vi "孔径结果转换.vi"(11 "Fitted Circle (Find Circular Edge 1)":T1 {"Average SNR (dB)" format="%.2f"; "Average Strength" format="%.2f"; "Roundness (Real-World)" format="%.2f"; "Radius (Real-World)" format="%.2f"; "Center (Real-World)"."Y" format="%.2f"; "Center (Real-World)"."X" format="%.2f"; "Radius (Pixels)" format="%.2f"; "Center (Pixels)"."Y" format="%.2f"; "Center (Pixels)"."X" format="%.2f"}) -> (3 "x+y":dbl format="%#_3f")   [LabVIEW 2017]
uses:
  Global System.vi
panel:
  out "F-格式字符串":string
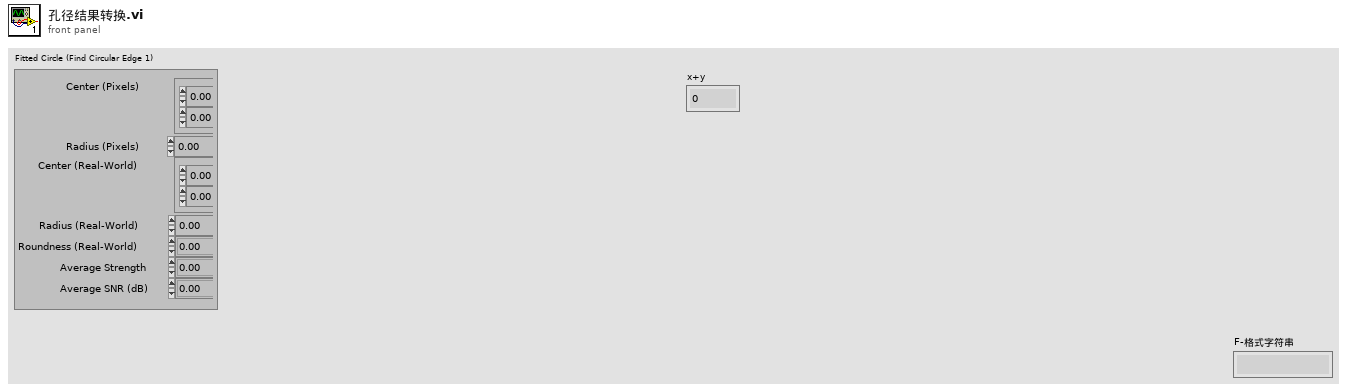
[diagram p1: front panel]
types:
  T1 = cluster{"Center (Pixels)":cluster{"X":sgl, "Y":sgl}, "Radius (Pixels)":dbl, "Center (Real-World)":cluster{"X":sgl, "Y":sgl}, "Radius (Real-World)":dbl, "Roundness (Real-World)":dbl, "Average Strength":dbl, "Average SNR (dB)":dbl}
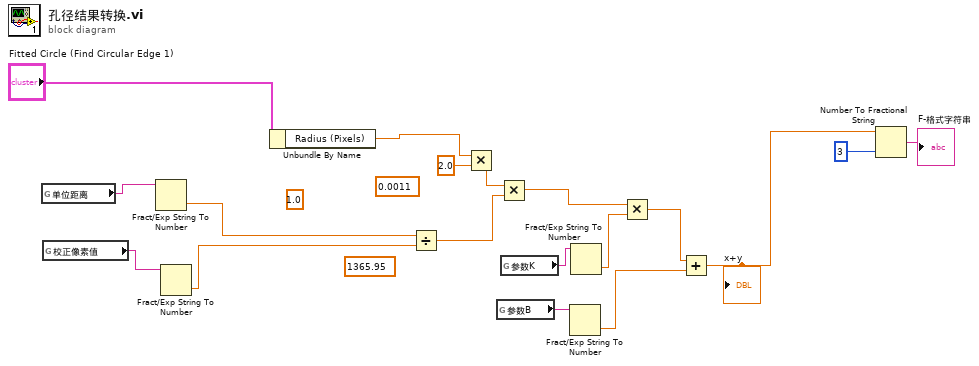
[diagram p0: block diagram]
diagram:
  (unwired) 1365.95 ("y")
  (unwired) 1.0 ("x")
  (unwired) 0.0011 ("y")
  n1 = global read "Global System.vi" "单位距离"() -> (w11:string)
  n2 = global read "Global System.vi" "校正像素值"() -> (w9:string)
  n3 = Fract/Exp String To Number(string=w11) -> (number=w10:dbl)  [unwired: 3 in, 1 out]
  n4 = Fract/Exp String To Number(string=w9) -> (number=w8:dbl)  [unwired: 3 in, 1 out]
  n5 = Unbundle By Name("Fitted Circle (Find Circular Edge 1)") -> ("Radius (Pixels)"=w14:dbl)
  n6 = Divide(x=w10, y=w8) -> (x/y=w12:dbl)
  n7 = Multiply(x=w14, y=2.0) -> (x*y=w15:dbl)
  n8 = global read "Global System.vi" "参数B"() -> (w6:string)
  n9 = Multiply(x=w15, y=w12) -> (x*y=w2:dbl)
  n10 = global read "Global System.vi" "参数K"() -> (w7:string)
  n11 = Fract/Exp String To Number(string=w6) -> (number=w3:dbl)  [unwired: 3 in, 1 out]
  n12 = Fract/Exp String To Number(string=w7) -> (number=w5:dbl)  [unwired: 3 in, 1 out]
  n13 = Multiply(x=w2, y=w5) -> (x*y=w4:dbl)
  n14 = Add(x=w4, y=w3) -> (x+y=w1:dbl)
  "x+y" <- w1
  n15 = Number To Fractional String(number=w1, precision (6)=i16 3 ("精度(6)")) -> (F-format string=→"F-格式字符串":string)  [unwired: 2 in]
